vi "Calculate Power.vi"(0 "input data":cdb[](array[numeric]), 13 "IQ rate":dbl=3072000000.0 format="%#_13p") -> (4 "time domain power output":waveform(dbl)(graph))   [LabVIEW 2019]
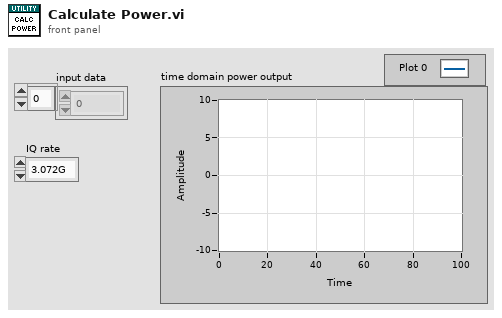
[diagram p1: front panel]
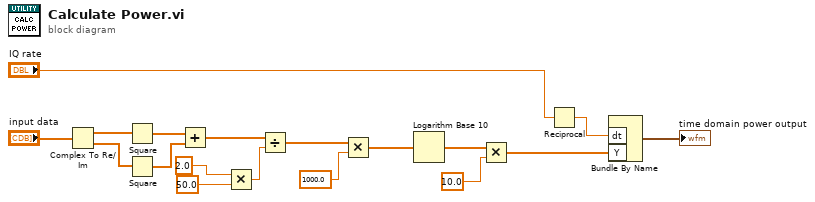
[diagram p0: block diagram]
diagram:
  n1 = Complex To Re/Im(x + iy="input data") -> (x=w14:dbl[], y=w15:dbl[])
  n2 = Square(x=w14) -> (x^2=w11:dbl[])
  n3 = Square(x=w15) -> (x^2=w10:dbl[])
  n4 = Add(x=w11, y=w10) -> (x+y=w9:dbl[])
  n5 = Multiply(x=2.0, y=50.0) -> (x*y=w8:dbl)
  n6 = Divide(x=w9, y=w8) -> (x/y=w5:dbl[])
  n7 = Multiply(x=w5, y=1000.0) -> (x*y=w3:dbl[])
  n8 = Logarithm Base 10(1:w3) -> (0:w2:dbl[])
  n9 = Multiply(x=w2, y=10.0) -> (x*y=w18:dbl[])
  n10 = Reciprocal(x="IQ rate") -> (1/x=w17:dbl)
  n11 = Bundle By Name("dt"=w17, "Y"=w18) -> (→"time domain power output":waveform(dbl))  [unwired: 1 in]
